vi "异步调用趋势图.vi"(9 "参数":string, 10 "Array输入":refnum<vi>, 11 "原点":T1) -> ()   [LabVIEW 2016, in "多参数状态显示.xctl"]
uses:
  <vilib>/Utility/miscctls.llb/LVPointTypeDef.ctl
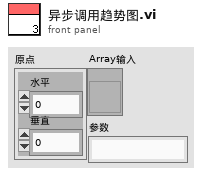
[diagram p1: front panel]
types:
  T1 = typedef "LVPointTypeDef.ctl" = cluster{"Horizontal":i16, "Vertical":i16}
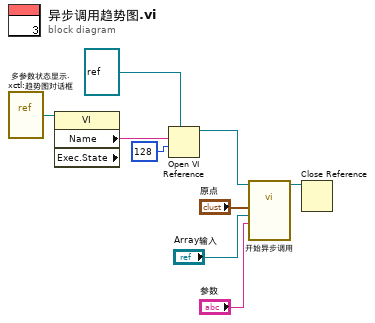
[diagram p0: block diagram]
diagram:
  n1 = vi-ref "多参数状态显示.xctl:趋势图对话框.vi"() -> (w8:refnum<vi>)
  n2 = property class="VI" props=["Name", "Exec.State"](reference=w8) -> ("Name"=w9:string)  [unwired: 1 in, 3 out]
  n3 = Open VI Reference(type specifier VI Refnum (for type only)=refnum<vi> refnum, vi path=w9, options=128 ("选项")) -> (vi reference=w6:refnum<vi>)  [unwired: 3 in, 1 out]
  n4 = call-by-ref "开始异步调用"(reference=w6, "参数"="参数", "Array输入"="Array输入", "原点"="原点") -> (reference out=w5:refnum<vi>)  [unwired: 10 in, 1 out]
  n5 = Close Reference(reference=w5) -> ()  [unwired: 1 in, 1 out]
